vi "GetFirmwareInfo.vi"(7 "LabVIEW Web Service Request":refnum<class "Web Request.lvclass">) -> ()   [LabVIEW 2017]
uses:
  <vilib>/wsapi/Web Request.lvclass
  <vilib>/addons/SystemInfoProcess/SystemInfoProcess.lvlib
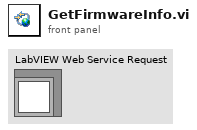
[diagram p1: front panel]
types:
  T1 = typedef "PointValueMap.lvlib/PointMap.ctl" = refnum<data-value>
  T2 = typedef "SystemInfoProcess.lvlib/ImageMetadata.ctl" = cluster{"Title":string, "Description":string, "ID":string, "Version":string}
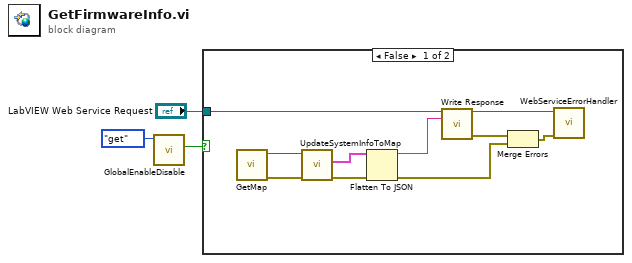
[diagram p0: block diagram]
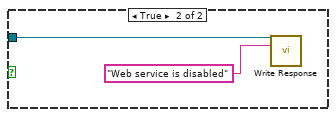
[diagram p2: hidden frame]
diagram:
  n1 = call "GlobalEnableDisable.vi"("action"=enum16{"init", "set", "get"}."get") -> ("DisableDeviceWebService"=w1:bool)  [unwired: 10 in]
  n2 = case shown="False" w1 {
    tunnel: "LabVIEW Web Service Request" -> [w13 w14]
    frame False {
      n3 = call <vilib>:"GetMap.vi"() -> ("error out"=w7:errorcluster, "SystemInfoMap"=w9:T1)  [unwired: 10 in]
      n4 = call <vilib>:"UpdateSystemInfoToMap.vi"("error in (no error)"=w7, "map in"=w9) -> ("error out"=w6:errorcluster, "system info"=w8:T2)  [unwired: 5 in, 3 out]
      n5 = Flatten To JSON(anything=w8, error in (no error)=w6) -> (JSON string=w12:string, 11:w4:errorcluster)  [unwired: 1 in]
      n6 = call <vilib>:"Write Response.vi"("LabVIEW Web Service Request"=w13, "response string"=w12) -> ("LabVIEW Web Service Request out"=w11:refnum<class "Web Request.lvclass">, "error out"=w10:errorcluster)  [unwired: 12 in]
      n7 = Merge Errors(w10, w4) -> (w5:errorcluster)
      n8 = call "WebServiceErrorHandler.vi"("LabVIEW Web Service Request"=w11, "error in (no error)"=w5) -> ()  [unwired: 12 in, 2 out]
    }
    frame True {
      n9 = call <vilib>:"Write Response.vi"("LabVIEW Web Service Request"=w14, "response string"="Web service is disabled") -> ()  [unwired: 12 in, 2 out]
    }
  }
